vi "BRig_Host_comm_tcp_parseCmd__getType.vi"(0 "input_strCmd":string, 2 "input_countCmd":i32, 6 "input_I_Stop":bool, 8 "input_I_ExpRun":bool) -> (10 "output_I_ExpRun":bool, 12 "output_I_Stop":bool, 14 "output_strType":u8)   [LabVIEW 2014]
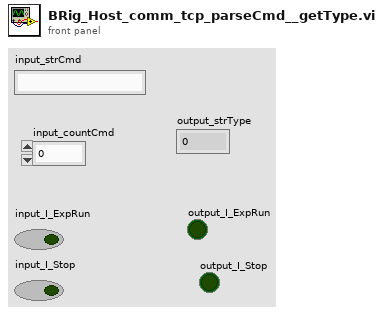
[diagram p1: front panel]
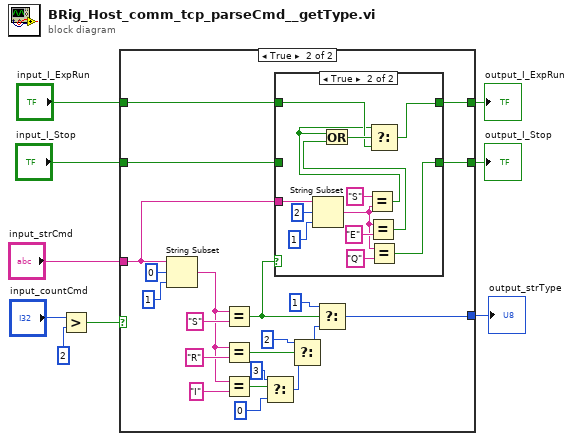
[diagram p0: block diagram]
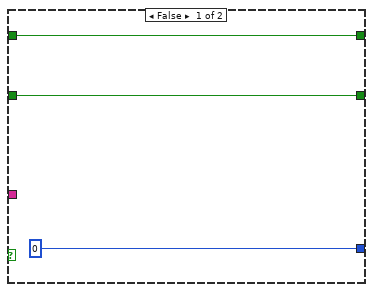
[diagram p2: hidden frame]
diagram:
  n1 = Greater?(x="input_countCmd", y=2) -> (0:w7:bool)
  n2 = case shown="True" w7 {
    tunnel: "input_strCmd" -> [_ w13]
    tunnel: [u8 0 ("t") w22] -> w6
    tunnel: "input_I_Stop" -> [w11 w17]
    tunnel: [w11 w14] -> w1
    tunnel: "input_I_ExpRun" -> [w10 w16]
    tunnel: [w10 w15] -> w2
    frame False {
    }
    frame True {
      n3 = String Subset(string=w13, offset (0)=0, length (rest)=1 ("length (rest)")) -> (substring=w18:string)
      n4 = Equal?(x=w18, y="S") -> (x = y?=w19:bool)
      n5 = Equal?(x=w18, y="R") -> (x = y?=w20:bool)
      n6 = Equal?(x=w18, y="I") -> (x = y?=w28:bool)
      n7 = Select(t=u8 3, s=w28, f=u8 0) -> (s? t:f=w25:u8)
      n8 = case shown="True" w19 {
        tunnel: w17 -> [w34 _]
        tunnel: w16 -> [w35 w40]
        tunnel: [w35 w39] -> w15
        tunnel: [w34 w42] -> w14
        tunnel: w13 -> [_ w36]
        frame False {
        }
        frame True {
          n9 = String Subset(string=w36, offset (0)=2, length (rest)=1 ("length (rest)")) -> (substring=w44:string)
          n10 = Equal?(x="S" ("y"), y=w44) -> (x = y?=w38:bool)
          n11 = Equal?(x=w44, y="E") -> (x = y?=w37:bool)
          n12 = Or(x=w38, y=w37) -> (x .or. y?=w41:bool)
          n13 = Select(t=w38, s=w41, f=w40) -> (s? t:f=w39:bool)
          n14 = Equal?(x=w44, y="Q") -> (x = y?=w42:bool)
        }
      }
      n15 = Select(t=u8 2, s=w20, f=w25) -> (s? t:f=w23:u8)
      n16 = Select(t=u8 1, s=w19, f=w23) -> (s? t:f=w22:u8)
    }
  }
  "output_strType" <- w6
  "output_I_ExpRun" <- w2
  "output_I_Stop" <- w1
